vi "Generate Initial Solution.vi"(8 "error in (no error)":errorcluster, 9 "seed":i32=-1, 10 "OSSP_Problem In":refnum<class "OSSP_Problem.lvclass">, 11 "SA in":refnum<class "SA.lvclass">) -> (0 "error out":errorcluster, 3 "SA out":refnum<class "SA.lvclass">)   [LabVIEW 2013, in "SA.lvclass"]
uses:
  SA.lvclass
  OSSP_Problem.lvclass
  SA.lvclass/SA.ctl
  <vilib>/Analysis/1siggen.llb/Riffle Array (I32).vi
  <vilib>/Analysis/NI_AALBase.lvlib
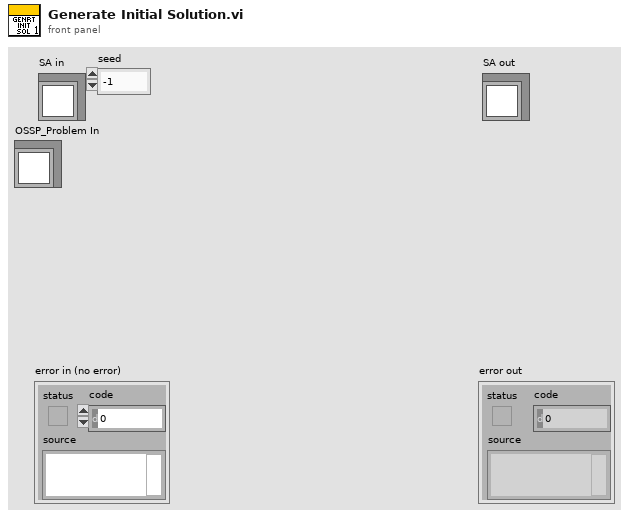
[diagram p1: front panel]
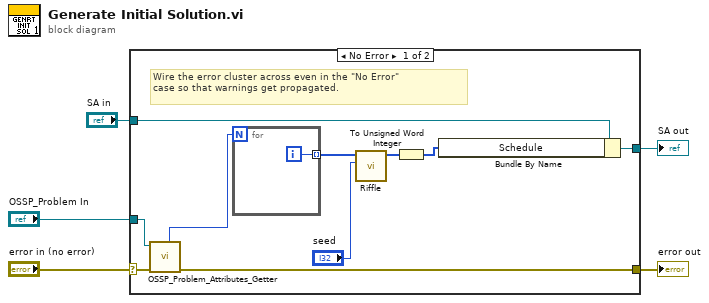
[diagram p0: block diagram]
diagram:
  n1 = case shown="No Error" "error in (no error)" {
    selector: "error in (no error)" -> [w7 w18]
    tunnel: [w6 w18] -> w4
    tunnel: [w10 w17] -> w2
    tunnel: "SA in" -> [w11 w17]
    tunnel: "OSSP_Problem In" -> [w15 _]
    frame No Error {
      # "Wire the error cluster across even in the \"No Error\"\ncase so that warnings get propagated."
      n2 = call "OSSP_Problem_Attributes_Getter.vi"("error in (no error)"=w7, "OSSP_Problem in"=w15) -> ("error out"=w6:errorcluster, "Dimension"=w14:i32)  [unwired: 3 in, 5 out]
      n3 = for {
        N: w14 -> [_]
        tunnel: [w16] -> w13 mode=indexing
        i -> [w16]
      }
      n4 = call-poly <vilib>:"Riffle.vi"("seed"="seed", "X"=w13) -> ("Riffled {X}"=w9:i32[])  [unwired: 7 in, 2 out]
      n5 = To Unsigned Word Integer(number=w9) -> (unsigned 16bit integer=w8:u16[])
      n6 = Bundle By Name(cluster=w11, "Schedule"=w8) -> (w10:refnum<class "SA.lvclass">)
    }
    frame Error {
    }
  }
  "error out" <- w4
  "SA out" <- w2
